vi "Visit_Source.vi"(8 "error in (no error)":errorcluster, 10 "address":string, 11 "Installer in":refnum<class "Installer.lvclass">) -> (0 "error out":errorcluster, 1 "source":refnum<class "IB_Source.lvclass">, 2 "address out":string, 3 "Installer out":refnum<class "Installer.lvclass">)   [LabVIEW 2020, in "Installer.lvclass"]
uses:
  <vilib>/AppBuilder/IB_Classes/Installer/Installer.lvclass
  <vilib>/AppBuilder/IB_Classes/Installer/Installer.lvclass/Installer.ctl
  <vilib>/AppBuilder/IB_Classes/Source/IB_Source.lvclass
  <vilib>/AppBuilder/IB_Classes/Source/Container/IB_Source_Container.lvclass
  <vilib>/AppBuilder/IB_Classes/Source/File/CtrFile/IB_CtrFile.lvclass
  e:/builds/penguin/labview/branches/2020/dev/dist/vi.lib/AppBuilder/IB_Classes/Source/File/IB_Source_File.lvclass
  e:/builds/penguin/labview/branches/2020/dev/dist/vi.lib/AppBuilder/IB_Classes/Source/IB_Source.lvclass
  e:/builds/penguin/labview/branches/2020/dev/dist/vi.lib/AppBuilder/IB_Classes/Source/File/CtrFile/IB_CtrFile.lvclass
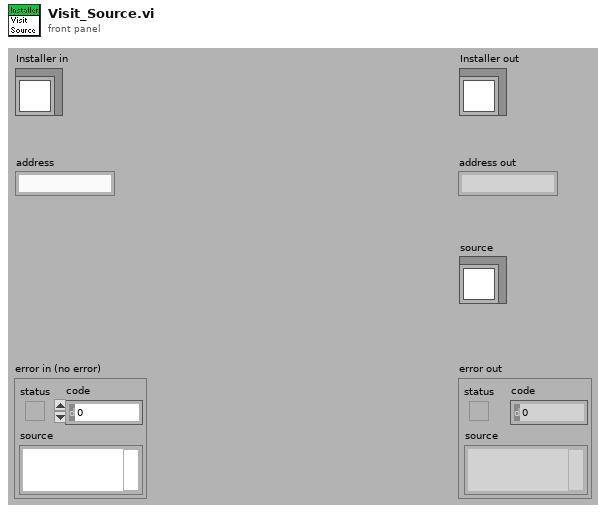
[diagram p1: front panel]
types:
  T1 = typedef "IB_Source.ctl" = cluster{"name":string, "sourceTag":string, "destTag":string, "path":path, "eng_installPath":string, "UI_inBuild?":bool, "str ref?":bool}
  T2 = typedef "IB_Source_Container.ctl" = cluster{"files":refnum<class "IB_CtrFile.lvclass">[], "previewed?":bool, "preview error?":bool}
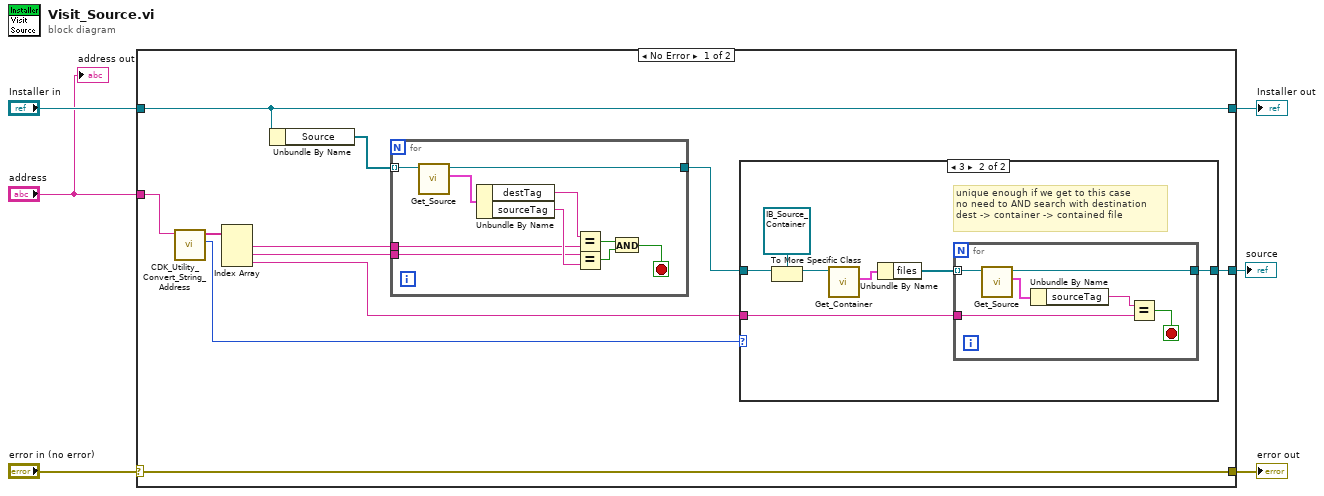
[diagram p0: block diagram]
diagram:
  n1 = case shown="No Error" "error in (no error)" {
    selector: "error in (no error)" -> [w17 w43]
    tunnel: [w17 w43] -> w5
    tunnel: [w16 w42] -> w3
    tunnel: "Installer in" -> [w16 w42]
    tunnel: "address" -> [w10 _]
    tunnel: [w11 _] -> w2
    frame No Error {
      n2 = call <resource>:"CDK_Utility_Convert_String_Address.vi"("address"=w10) -> ("address size"=w8:i32, "address parts"=w9:string[])  [unwired: 9 out]
      n3 = Index Array(array=w9) -> (element #1=w7:string, element #2=w14:string, element #3=w12:string)  [unwired: 3 in]
      n4 = Unbundle By Name(w16) -> ("Source"=w15:refnum<class "IB_Source.lvclass">[])
      n5 = for {
        tunnel: w15 -> [w41] mode=indexing
        tunnel: w14 -> [w33]
        tunnel: [w40] -> w13
        tunnel: w7 -> [w34]
        stop <- w32 stop-if-true
        n6 = call <vilib>:"Get_Source.vi"("IB_Source in"=w41) -> ("data"=w35:T1, "IB_Source out"=w40:refnum<class "IB_Source.lvclass">)  [unwired: 1 in, 8 out]
        n7 = Unbundle By Name(w35) -> ("destTag"=w36:string, "sourceTag"=w37:string)
        n8 = Equal?(x=w36, y=w34) -> (x = y?=w38:bool)
        n9 = Equal?(x=w33, y=w37) -> (x = y?=w39:bool)
        n10 = And(x=w38, y=w39) -> (x .and. y?=w32:bool)
      }
      n11 = case shown="3" w8 {
        tunnel: w13 -> [w18 w24]
        tunnel: w12 -> [_ w20]
        tunnel: [w18 w19] -> w11
        frame 2, Default {
        }
        frame 3 {
          # "unique enough if we get to this case\nno need to AND search with destination\ndest -> container -> contained file"
          n12 = To More Specific Class(target class=refnum<class "IB_Source_Container.lvclass"> refnum ("IB_Source_Container.lvclass"), reference=w24) -> (specific class reference=w23:refnum<class "IB_Source_Container.lvclass">)  [unwired: 1 in, 1 out]
          n13 = call <vilib>:"Get_Container.vi"("IB_Source_Container in"=w23) -> ("data"=w22:T2)  [unwired: 1 in, 9 out]
          n14 = Unbundle By Name(w22) -> ("files"=w21:refnum<class "IB_CtrFile.lvclass">[])
          n15 = for {
            tunnel: w21 -> [w31] mode=indexing
            tunnel: w20 -> [w29]
            tunnel: [w27] -> w19
            stop <- w26 stop-if-true
            n16 = call <vilib>:"Get_Source.vi"("IB_Source in"=w31) -> ("data"=w28:T1, "IB_Source out"=w27:refnum<class "IB_CtrFile.lvclass">)  [unwired: 1 in, 8 out]
            n17 = Unbundle By Name(w28) -> ("sourceTag"=w30:string)
            n18 = Equal?(x=w30, y=w29) -> (x = y?=w26:bool)
          }
        }
      }
    }
    frame Error {
    }
  }
  "error out" <- w5
  "Installer out" <- w3
  "source" <- w2
  "address out" <- "address"
